vi "Verbose Mode.vi"() -> ()   [LabVIEW 2021, in "Notebook.lvlib"]
uses:
  Notebook.lvlib
panel:
  out "Verbose Error Mode":bool
  out "Verbose Mode":bool
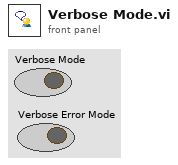
[diagram p1: front panel]
diagram:
